vi "ZREAD CAM.vi"() -> ()   [LabVIEW 2014]
uses:
  <vilib>/userdefined/High Color/IMAQdx.ctl
  <vilib>/vision/driver/NI_Vision_Acquisition_Software.lvlib
panel:
  out "Image":T1(plugin-control)
  in  "Session In":T2
  in  "stop":bool
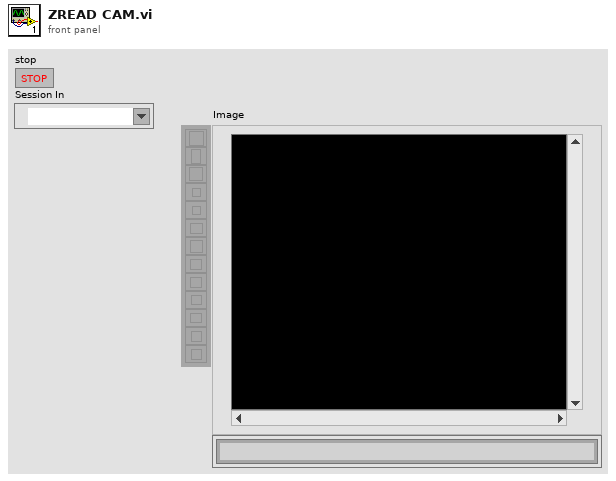
[diagram p1: front panel]
types:
  T1 = typedef "IMAQ Image.ctl" = refnum<image>
  T2 = typedef "IMAQdx.ctl" = refnum<k21>
  T3 = typedef "Image Type" = u32
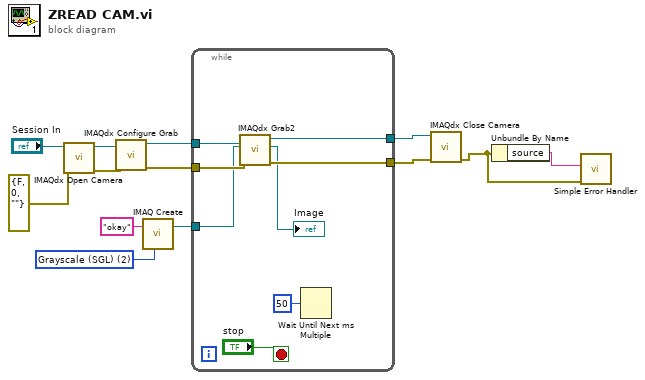
[diagram p0: block diagram]
diagram:
  w4 = T3 2 items=["Grayscale (U8)", "Grayscale (I16)", "Grayscale (SGL)", "Complex (CSG)", "RGB (U32)", "HSL (U32)", "RGB (U64)", "Grayscale (U16)"] ("Image Type")
  n1 = call <vilib>:"IMAQdx Open Camera.vi"("error in"=errorcluster {"status"=FALSE, "code"=0, "source"=""}, "Session In"="Session In") -> ("error out"=w8:errorcluster, "Session Out"=w9:T2)  [unwired: 8 in]
  n2 = call <vilib>:"IMAQdx Configure Grab.vi"("error in"=w8, "Session In"=w9) -> ("error out"=w13:errorcluster, "Session Out"=w12:T2)  [unwired: 8 in]
  n3 = call "IMAQ Create"("Image Name"="okay", "Image Type"=w4) -> ("New Image"=w3:T1)  [unwired: 3 in, 1 out]
  n4 = while {
    tunnel: w13 -> [w21]
    tunnel: w12 -> [w20]
    tunnel: [w18] -> w7
    tunnel: [w17] -> w6
    tunnel: w3 -> [w16]
    stop <- "stop" stop-if-true
    n5 = call <vilib>:"IMAQdx Grab2.vi"("error in"=w21, "Image In"=w16, "Session In"=w20) -> ("error out"=w17:errorcluster, "Image Out"=→"Image":T1, "Session Out"=w18:T2)  [unwired: 5 in, 1 out]
    n6 = Wait Until Next ms Multiple(millisecond multiple=u32 50) -> ()  [unwired: 1 out]
  }
  n7 = call <vilib>:"IMAQdx Close Camera.vi"("error in"=w6, "Session In"=w7) -> ("error out"=w2:errorcluster)  [unwired: 9 in]
  n8 = Unbundle By Name(w2) -> ("source"=w1:string)
  n9 = call <vilib>:"Simple Error Handler.vi"("error source (\" \")"=w1, "error in (no error)"=w2) -> ()  [unwired: 3 in, 5 out]
